vi "ParameterInsert.vi"(4 "result":string, 6 "unit":string, 7 "productsName":string, 8 "limitL":dbl=nan, 9 "limitH":dbl=nan, 10 "notes":string, 11 "parameterName":string) -> ()   [LabVIEW 2013]
uses:
  <vilib>/Utility/VariantDataType/Type.ctl
  <vilib>/Utility/VariantDataType/VariantType.lvlib
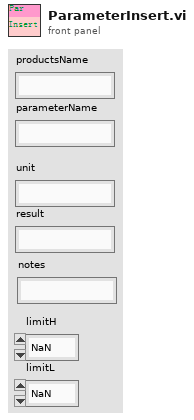
[diagram p1: front panel]
types:
  T1 = typedef "VariantType.lvlib/Type.ctl" = enum8{"Invalid Type", "Void", "I8", "I16", "I32", "I64", "U8", "U16", "U32", "U64", "Single Float", "Double Float", "Extended Float", "Single Complex", "Double Complex", "Extended Complex", "Enum U8", "Enum U16", "Enum U32", "Enum U64", "Single Float With Unit", "Double Float With Unit", "Extended Float With Unit", "Single Complex with Unit", "Double Complex with Unit", "Extended Complex with Unit", "Boolean", "String", "Path", "Picture", "Tag", "Array", "Cluster", "Variant", "LV Variant", "Waveform", "Timestamp", "Digital Waveform", "Digital Data", "ExpressData", "Refnum", "External Data", "VI", "Poly VI", "LabVIEW Class Instance", "Fixed Point"}
  T2 = cluster{"Type Enum":T1, "标签.文本":string, "productsName":string}
  T3 = cluster{"Type Enum":T1, "标签.文本":string, "parameterName":string}
  T4 = cluster{"Type Enum":T1, "标签.文本":string, "unit":string}
  T5 = cluster{"Type Enum":T1, "标签.文本":string, "result":string}
  T6 = cluster{"Type Enum":T1, "标签.文本":string, "notes":string}
  T7 = cluster{"Type Enum":T1, "标签.文本":string, "notes":string}[]
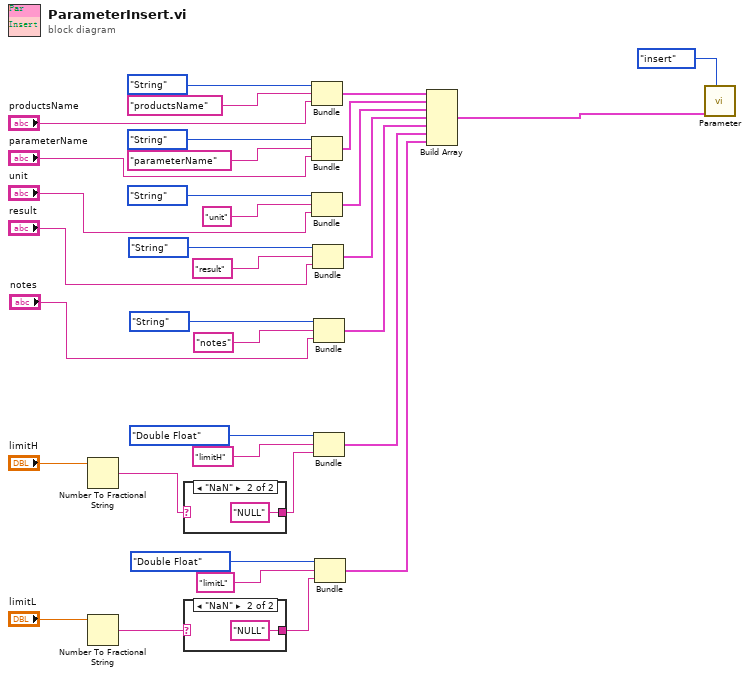
[diagram p0: block diagram]
diagram:
  n1 = Number To Fractional String(number="limitH") -> (F-format string=w9:string)  [unwired: 3 in]
  n2 = Number To Fractional String(number="limitL") -> (F-format string=w12:string)  [unwired: 3 in]
  n3 = case shown="\"NaN\"" w9 {
    selector: w9 -> [w35 _]
    tunnel: [w35 "NULL"] -> w8
    frame "假", Default {
    }
    frame "NaN" {
    }
  }
  n4 = case shown="\"NaN\"" w12 {
    selector: w12 -> [w37 _]
    tunnel: [w37 "NULL"] -> w11
    frame "假", Default {
    }
    frame "NaN" {
    }
  }
  n5 = Bundle("Type Enum"=Type."String", "标签.文本"="productsName", "productsName"="productsName") -> (w34:T2)  [unwired: 1 in]
  n6 = Bundle("Type Enum"=Type."String", "标签.文本"="parameterName", "parameterName"="parameterName") -> (w17:T3)  [unwired: 1 in]
  n7 = Bundle("Type Enum"=Type."String", "标签.文本"="unit", "unit"="unit") -> (w16:T4)  [unwired: 1 in]
  n8 = Bundle("Type Enum"=Type."String", "标签.文本"="result", "result"="result") -> (w15:T5)  [unwired: 1 in]
  n9 = Bundle("Type Enum"=Type."String", "标签.文本"="notes", "notes"="notes") -> (w1:T6)  [unwired: 1 in]
  n10 = Bundle("Type Enum"=Type."Double Float", "标签.文本"="limitH", w8) -> (w2:cluster{"Type Enum":T1, "标签.文本":string, string})  [unwired: 1 in]
  n11 = Bundle("Type Enum"=Type."Double Float", "标签.文本"="limitL", w11) -> (w3:cluster{"Type Enum":T1, "标签.文本":string, string})  [unwired: 1 in]
  n12 = Build Array(w34, w17, w16, w15, w1, w2, w3) -> (w10:T7)
  n13 = call "Parameter.vi"("模式"=enum16{"select", "insert", "update", "delete"}."insert", "nameData"=w10) -> ()  [unwired: 9 in, 1 out]
